vi "Gen NtripClient TCP command.vi"() -> ()   [LabVIEW 2019]
uses:
  Ctrl/Ntrip_Account_db.ctl
panel:
  in  "Current Ntrip account":T1={"address"="gnss.eseoul.go.kr", "port "=2101, "id"="seoul", "pwd"="seoul", "ref pt"="YONS-RTCM32-M5"}
  in  "cmd":enum16{"Get ref", "Get rtcm"}(ring)
  out "ascii":string
  out "hex":string
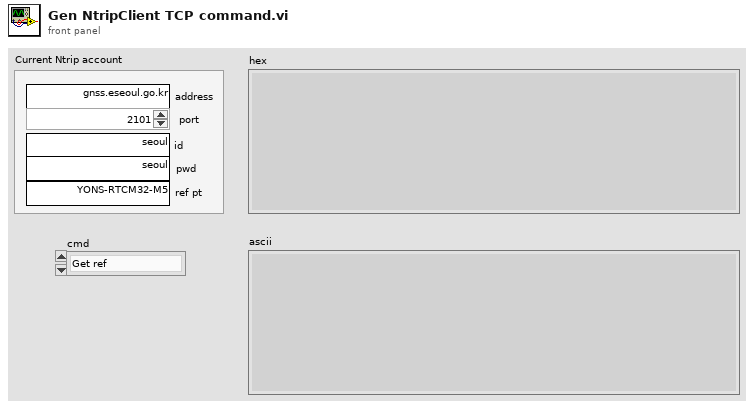
[diagram p1: front panel]
types:
  T1 = typedef "Ntrip_Account_db.ctl" = cluster{"address":string, "port ":u16, "id":string, "pwd":string, "ref pt":string}
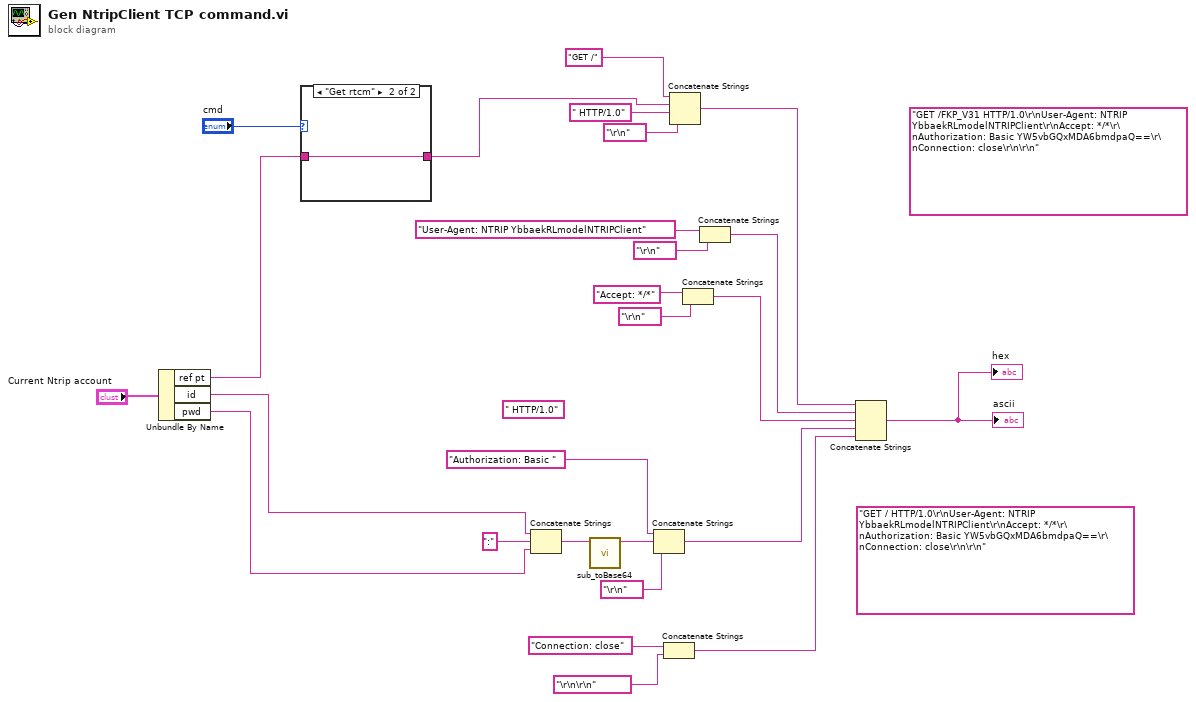
[diagram p0: block diagram]
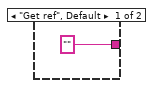
[diagram p2: hidden frame]
diagram:
  (unwired) "GET /FKP_V31 HTTP/1.0\r\nUser-Agent: NTRIP YbbaekRLmodelNTRIPClient\r\nAccept: */*\r\nAuthorization: Basic YW5vbGQxMDA6bmdpaQ==\r\nConnection: close\r\n\r\n" ("ascii 2")
  (unwired) "GET / HTTP/1.0\r\nUser-Agent: NTRIP YbbaekRLmodelNTRIPClient\r\nAccept: */*\r\nAuthorization: Basic YW5vbGQxMDA6bmdpaQ==\r\nConnection: close\r\n\r\n" ("ascii 2")
  (unwired) " HTTP/1.0" ("string")
  n1 = Unbundle By Name("Current Ntrip account") -> ("ref pt"=w17:string, "id"=w25:string, "pwd"=w26:string)
  n2 = case shown="\"Get rtcm\"" "cmd" {
    tunnel: w17 -> [_ w28]
    tunnel: ["" ("문자열") w28] -> w1
    frame "Get ref", Default {
    }
    frame "Get rtcm" {
    }
  }
  n3 = Concatenate Strings(w25, ":" ("string"), w26) -> (w24:string)
  n4 = call "sub_toBase64.vi"("str-in"=w24) -> ("Base64"=w20:string)  [unwired: 10 in]
  n5 = Concatenate Strings("Authorization: Basic " ("data in"), w20, "\r\n" ("string")) -> (w22:string)
  n6 = Concatenate Strings("Connection: close" ("data in"), "\r\n\r\n" ("string")) -> (w2:string)
  n7 = Concatenate Strings("GET /" ("data in"), w1, " HTTP/1.0" ("string"), "\r\n" ("string")) -> (w12:string)
  n8 = Concatenate Strings("Accept: */*" ("data in"), "\r\n" ("string")) -> (w3:string)
  n9 = Concatenate Strings("User-Agent: NTRIP YbbaekRLmodelNTRIPClient" ("data in"), "\r\n" ("string")) -> (w4:string)
  n10 = Concatenate Strings(w12, w4, w3, w22, w2) -> (→"hex" →"ascii":string)
